vi "Launch Quad With Bells and Whistles.vi"   [LabVIEW 2015]
uses:
  ExampleSimpleRootModel/SimpleRootModel.lvclass
  TwoPaneViewManager/TwoPaneViewManager.lvclass
  SimpleViewModel/SimpleViewModel.lvclass
  Framework/Mediator/Mediator/Mediator.lvclass
  Framework/Mediator/MediatorBusMonitor/MediatorBusMonitor.lvclass
  <vilib>/ActorFramework/Message Enqueuer/Message Priority.ctl
  Framework/IViewable/IViewable/View Position Enum.ctl
  SimpleChart/SimpleChart.lvclass
  VerticalSlide/VerticalSlide.lvclass
  PauseResumeButtons/PauseResumeButtons.lvclass
  Framework/IViewManager/IViewManager Messages/Launch Nested Views Msg/Launch Nested Views Msg.lvclass/Launch Nested Views Msg.ctl
  Framework/IViewManager/IViewManager/IViewManager.lvclass/IViewManager.ctl
  Framework/IMediator/IMediator/IMediator.lvclass/IMediator.ctl
  Framework/IViewModel/IViewModel/IViewModel.lvclass/IViewModel.ctl
  Framework/IViewable/IViewable Messages/Open Front Panel Msg/Open Front Panel Msg.lvclass/Open Front Panel Msg.ctl
  <vilib>/ActorFramework/Message Enqueuer/Message Enqueuer.lvclass/Message Enqueuer.ctl
  Framework/IViewManager/IViewManager Messages/Launch Nested Views Msg/Pack Launch Nested Views Msg.vi
  Framework/IViewManager/IViewManager/Write Startup Launch Nested Views Msg.vi
  <vilib>/ActorFramework/Message Enqueuer/Enqueue.vi
  <vilib>/ActorFramework/Message Priority Queue/Priority Enqueue.vi
  Framework/IViewManager/IViewManager Messages/Launch Nested Views Msg/Launch Nested Views Msg.lvclass
  Framework/IViewable/IApplicationStyle/IApplicationStyle.lvclass
  Framework/IViewable/IViewable Messages/Open Front Panel Msg/Open Front Panel Msg.lvclass
  <vilib>/ActorFramework/Actor/Actor.lvclass
  Framework/IViewModel/IViewModel/IViewModel.lvclass
  Framework/IMediator/IMediator/IMediator.lvclass
  <vilib>/ActorFramework/Message Enqueuer/Message Enqueuer.lvclass
  Framework/IViewable/IViewable/IViewable.lvclass
  Framework/IViewManager/IViewManager/IViewManager.lvclass
  ViewManager/QuadViewManager/QuadViewManager.lvclass
panel:
  # "This example launches a QuadViewManager with other Viewables nested inside"
types:
  T1 = typedef "IViewable.lvlib/IViewable.lvclass/View Position Enum.ctl" = enum16{"Centered", "Maximized", "Minimized", "Custom", "Unchanged"}
  T2 = typedef "Actor Framework.lvlib/Message Enqueuer.lvclass/Message Priority.ctl" = enum16{"Low", "Normal", "High"}
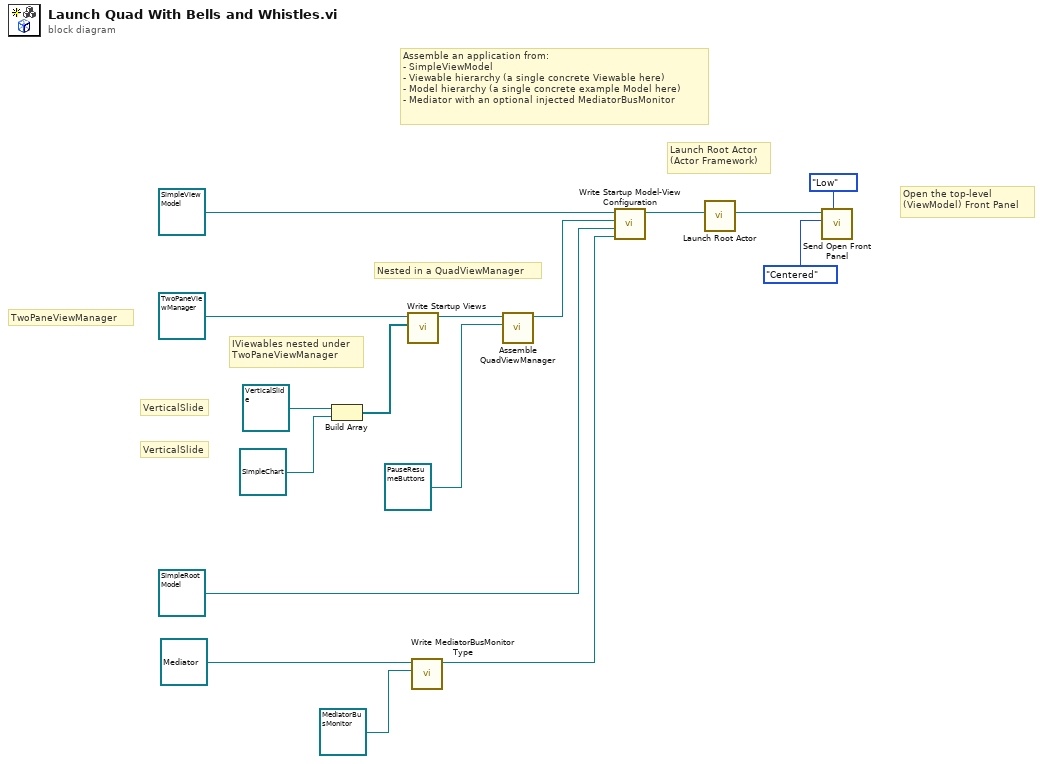
[diagram p0: block diagram]
diagram:
  # "Nested in a QuadViewManager"
  # "VerticalSlide"
  # "VerticalSlide"
  # "IViewables nested under \nTwoPaneViewManager"
  # "TwoPaneViewManager"
  # "Open the top-level\n(ViewModel) Front Panel"
  # "Launch Root Actor\n(Actor Framework)"
  # "Assemble an application from:\n- SimpleViewModel\n- Viewable hierarchy (a single concrete Viewable here)\n- Model hierarchy (a single concrete example Model here)\n- Mediator with an optional injected MediatorBusMonitor"
  n1 = Build Array(refnum<class "VerticalSlide.lvclass"> refnum ("MVAExamples.lvlib:VerticalSlide.lvclass"), refnum<class "SimpleChart.lvclass"> refnum ("MVAExamples.lvlib:SimpleChart.lvclass")) -> (w4:refnum<class "IViewable.lvclass">[])
  n2 = call "Write Startup Views.vi"("Startup Views"=w4, "IViewManager in"=refnum<class "TwoPaneViewManager.lvclass"> refnum ("MVAExamples.lvlib:TwoPaneViewManager.lvclass")) -> ("IViewManager out"=w3:refnum<class "TwoPaneViewManager.lvclass">)  [unwired: 9 in]
  n3 = call "Write MediatorBusMonitor Type.vi"("MediatorBusMonitor (Type)"=refnum<class "MediatorBusMonitor.lvclass"> refnum ("Mediator.lvlib:MediatorBusMonitor.lvclass"), "IMediator in"=refnum<class "Mediator.lvclass"> refnum ("Mediator.lvlib:Mediator.lvclass")) -> ("IMediator out"=w11:refnum<class "Mediator.lvclass">)  [unwired: 9 in]
  n4 = call "Assemble QuadViewManager.vi"("Top-Right View"=refnum<class "PauseResumeButtons.lvclass"> refnum ("MVAExamples.lvlib:PauseResumeButtons.lvclass"), "Top-Left View"=w3) -> ("QuadViewManager out"=w2:refnum<class "QuadViewManager.lvclass">)  [unwired: 9 in]
  n5 = call "Write Startup Model-View Configuration.vi"("Mediator Type"=w11, "Model Type"=refnum<class "SimpleRootModel.lvclass"> refnum ("MVAExamples.lvlib:SimpleRootModel.lvclass"), "Startup View Configuration"=w2, "IViewModel In"=refnum<class "SimpleViewModel.lvclass"> refnum ("MVAExamples.lvlib:SimpleViewModel.lvclass")) -> ("IViewModel Out"=w10:refnum<class "SimpleViewModel.lvclass">)  [unwired: 7 in]
  n6 = call <vilib>:"Launch Root Actor.vi"("Actor"=w10) -> ("Actor's Enqueuer"=w9:refnum<class "Message Enqueuer.lvclass">)  [unwired: 9 in, 1 out]
  n7 = call "Send Open Front Panel.vi"("Message Priority (Normal)"=Message_Priority."Low", "Position"=View_Position_Enum."Centered", "Message Enqueuer"=w9) -> ()  [unwired: 7 in, 2 out]
